vi "uTransport_DelayedSend.vi"(6 "# of times (1)":i32=1, 8 "error in (no error)":errorcluster, 9 "Delay (ms)":i32, 10 "Msg":refnum<class "uMsg.lvclass">, 11 "uTransport in":refnum<class "uTransport.lvclass">) -> (0 "error out":errorcluster, 3 "uMsg_Delayed out":refnum<class "uMsg_Delayed.lvclass">)   [LabVIEW 2023, in "uLib.lvlib" / "uTransport.lvclass"]
doc: "Send a delayed message on the transport.\nBy default, a single message will be sent after the specified delay. To send more than one message, wire in the '# of times' terminal. Wiring in 0 leads to this method not sending any messages out. Set to (-1) for infinite sending until the 'Abort Future Copies method is invoked' or the receiver uTransport becomes invalid, whichever occurs first."
uses:
  uTransport.lvclass
  uMsg/uMsg_Delayed/uMsg_Delayed.lvclass
  uMsg/uMsg/uMsg.lvclass
  uMsg/uMsg/uMsg.lvclass/uMsg.ctl
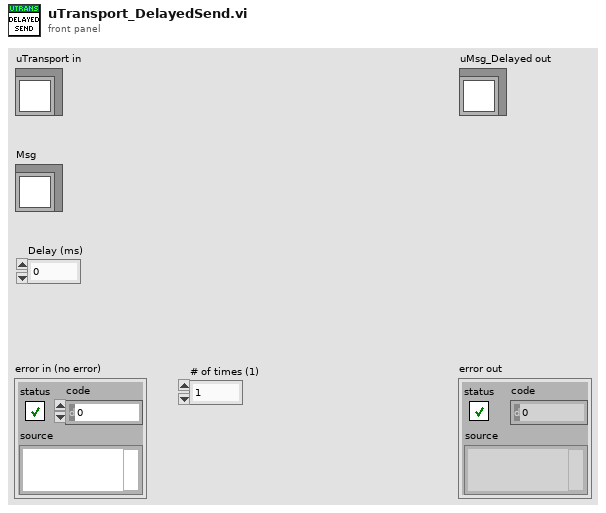
[diagram p1: front panel]
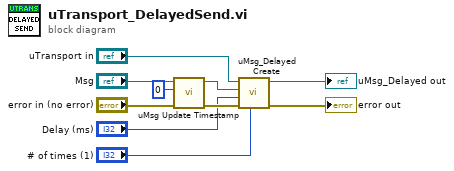
[diagram p0: block diagram]
diagram:
  n1 = call "uMsg Update Timestamp.vi"("error in (no error)"="error in (no error)", "Timestamp"=u32 0, "uMsg in"="Msg") -> ("error out"=w5:errorcluster, "uMsg out"=w7:refnum<class "uMsg.lvclass">)  [unwired: 7 in]
  n2 = call "uMsg_Delayed Create.vi"("# of times (1)"="# of times (1)", "error in (no error)"=w5, "delay (ms)"="Delay (ms)", "Msg"=w7, "Destination"="uTransport in") -> ("error out"=→"error out":errorcluster, "uMsg_Delayed out"=→"uMsg_Delayed out":refnum<class "uMsg_Delayed.lvclass">)  [unwired: 5 in]
